vi "SaveImage_single.vi"(8 "error in (no error)":errorcluster, 10 "base path":path, 11 "Image Src A":T1) -> (0 "error out":errorcluster)   [LabVIEW 2020]
uses:
  <vilib>/vision/NI_Vision_Development_Module.lvlib
  <vilib>/vision/Image Controls.llb/IMAQ Image.ctl
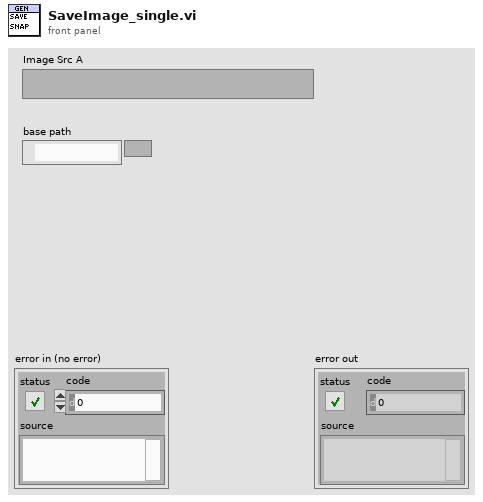
[diagram p1: front panel]
types:
  T1 = typedef "IMAQ Image.ctl" = refnum<image>
  T2 = typedef "Image Type" = u32
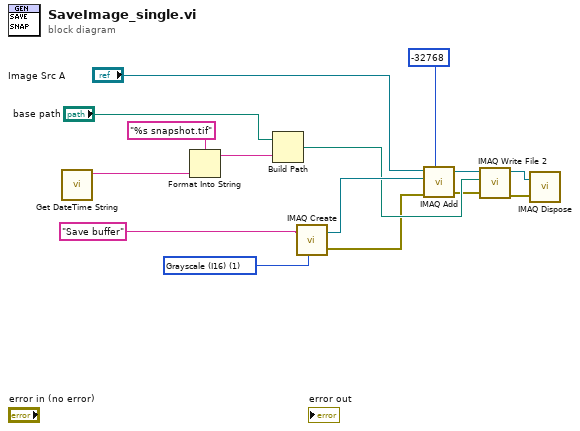
[diagram p0: block diagram]
diagram:
  w15 = T2 1 items=["Grayscale (U8)", "Grayscale (I16)", "Grayscale (SGL)", "Complex (CSG)", "RGB (U32)", "HSL (U32)", "RGB (U64)"] ("Image Type")
  n1 = call <userlib>:"Get DateTime String.vi"() -> ("date/time string"=w3:string)  [unwired: 10 in, 1 out]
  n2 = Format Into String(format string="%s snapshot.tif", w3) -> (resulting string=w12:string)  [unwired: 2 in, 1 out]
  n3 = Build Path(base path="base path", name or relative path=w12) -> (appended path=w13:path)
  n4 = call "IMAQ Create"("Image Name"="Save buffer" ("string"), "Image Type"=w15) -> ("New Image"=w14:T1, "error out"=w8:errorcluster)  [unwired: 3 in]
  n5 = call "IMAQ Add"("Image Src A"="Image Src A", "Constant"=i16 -32768, "Image Dst"=w14, "error in (no error)"=w8) -> ("Image Dst Out"=w11:T1, "error out"=w7:errorcluster)  [unwired: 3 in]
  n6 = call-poly "IMAQ Write File 2"("error in (no error)"=w7, "File Path"=w13, "Image"=w11) -> ("error out"=w9:errorcluster, "Image Out (duplicate)"=w10:T1)  [unwired: 7 in]
  n7 = call "IMAQ Dispose"("Image"=w10, "error in (no error)"=w9) -> ()  [unwired: 4 in, 1 out]
